vi "Configure Scan Monitor.vi"(0 "VISA resource name":refnum<visa-resource-name>, 1 "Lower (0)":dbl, 2 "Channel List Monitor (\"\")":string, 3 "Delay Seconds (0 s)":u32, 7 "Scan Mode (0: Off)":i32(ring) items=["Off", "Upper", "Lower", "Window"], 9 "Channel List Scan(\"\")":string, 11 "error in (no error)":errorcluster, 12 "Upper (0)":dbl, 13 "Reading Buffer (\"\")":string) -> (4 "VISA resource name out":refnum<visa-resource-name>, 15 "error out":errorcluster)   [LabVIEW 2023, in "Keithley DMM6500 DAQ6500 Series.lvlib"]
doc: "Configures the route scan monitor."
uses:
  <instrlib>/Keithley DMM6500 DAQ6500 Series/Keithley DMM6500 DAQ6500 Series.lvlib
  <vilib>/Utility/error.llb/Trim Whitespace One-Sided.vi
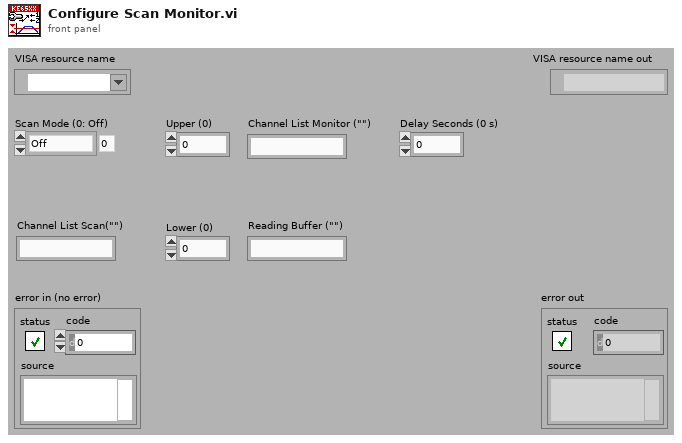
[diagram p1: front panel]
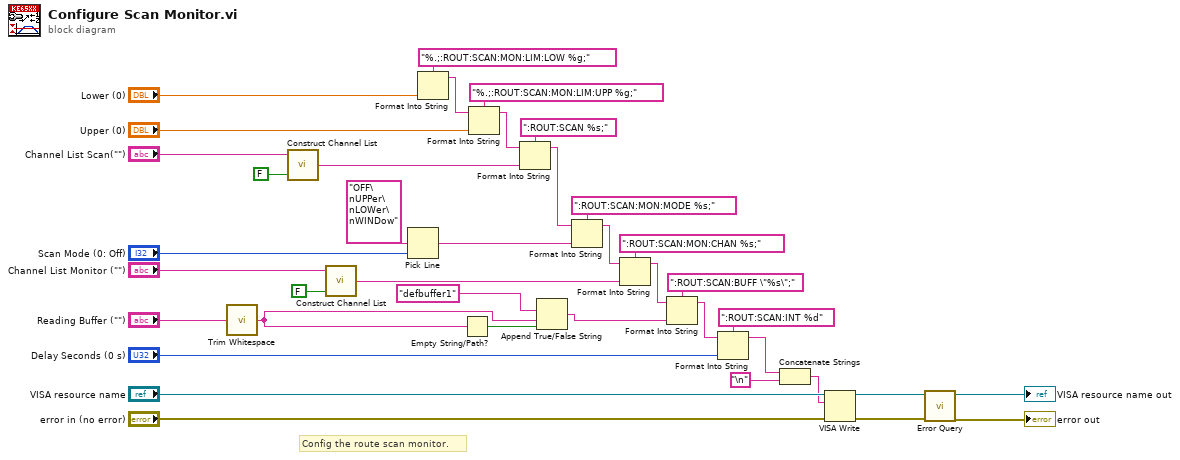
[diagram p0: block diagram]
diagram:
  # "Config the route scan monitor."
  n1 = call <vilib>:"Trim Whitespace.vi"("string"="Reading Buffer (\"\")") -> ("trimmed string"=w1:string)  [unwired: 1 in]
  n2 = call <instrlib>:"Construct Channel List.vi"("Add Comma (True)"=FALSE, "Channel List"="Channel List Scan(\"\")") -> ("Channel List String"=w19:string)  [unwired: 1 in]
  n3 = call <instrlib>:"Construct Channel List.vi"("Add Comma (True)"=FALSE, "Channel List"="Channel List Monitor (\"\")") -> ("Channel List String"=w17:string)  [unwired: 1 in]
  n4 = Pick Line(multi-line string="OFF\nUPPer\nLOWer\nWINDow", line index="Scan Mode (0: Off)") -> (output string=w10:string)  [unwired: 1 in]
  n5 = Format Into String(format string="%.;:ROUT:SCAN:MON:LIM:LOW %g;", "Lower (0)") -> (resulting string=w11:string)  [unwired: 2 in, 1 out]
  n6 = Empty String/Path?(string/path=w1) -> (empty?=w5:bool)
  n7 = Format Into String(format string="%.;:ROUT:SCAN:MON:LIM:UPP %g;", initial string=w11, "Upper (0)") -> (resulting string=w32:string)  [unwired: 1 in, 1 out]
  n8 = Format Into String(format string=":ROUT:SCAN %s;", initial string=w32, w19) -> (resulting string=w15:string)  [unwired: 1 in, 1 out]
  n9 = Append True/False String(1:w5, 2:w1, 3:"defbuffer1" ("true string")) -> (0:w3:string)  [unwired: 1 in]
  n10 = Format Into String(format string=":ROUT:SCAN:MON:MODE %s;", initial string=w15, w10) -> (resulting string=w14:string)  [unwired: 1 in, 1 out]
  n11 = Format Into String(format string=":ROUT:SCAN:MON:CHAN %s;", initial string=w14, w17) -> (resulting string=w13:string)  [unwired: 1 in, 1 out]
  n12 = Format Into String(format string=":ROUT:SCAN:BUFF \"%s\";", initial string=w13, w3) -> (resulting string=w30:string)  [unwired: 1 in, 1 out]
  n13 = Format Into String(format string=":ROUT:SCAN:INT %d", initial string=w30, "Delay Seconds (0 s)") -> (resulting string=w12:string)  [unwired: 1 in, 1 out]
  n14 = Concatenate Strings(w12, "\n") -> (w21:string)
  n15 = VISA Write(VISA resource name="VISA resource name", write buffer=w21, error in (no error)="error in (no error)") -> (VISA resource name out=w25:refnum<visa-resource-name>, error out=w24:errorcluster)  [unwired: 1 out]
  n16 = call <instrlib>:"Error Query.vi"("error in (no error)"=w24, "VISA resource name"=w25) -> ("error out"=→"error out":errorcluster, "VISA resource name out"=→"VISA resource name out":refnum<visa-resource-name>)  [unwired: 6 in, 2 out]
